vi "콜라자판기.vi"() -> ()   [LabVIEW 2014]
panel:
  out "그림 링":u16(ring)
  in  "종료":bool
  in  "반환":bool
  in  "구매":bool
  out "투입금액형":i32
  in  "동전":T1
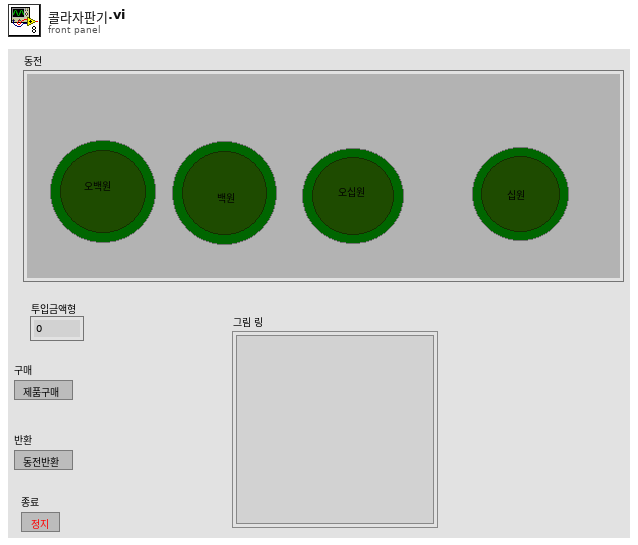
[diagram p1: front panel]
types:
  T1 = cluster{"오백원":bool, "백원":bool, "오십원":bool, "십원":bool}
  T2 = typedef "자판기.ctl" = enum16{"idle", "초기화", "종료", "구매", "반환"}
  T3 = enum8{"Enabled", "Disabled", "Disabled and Grayed Out"}
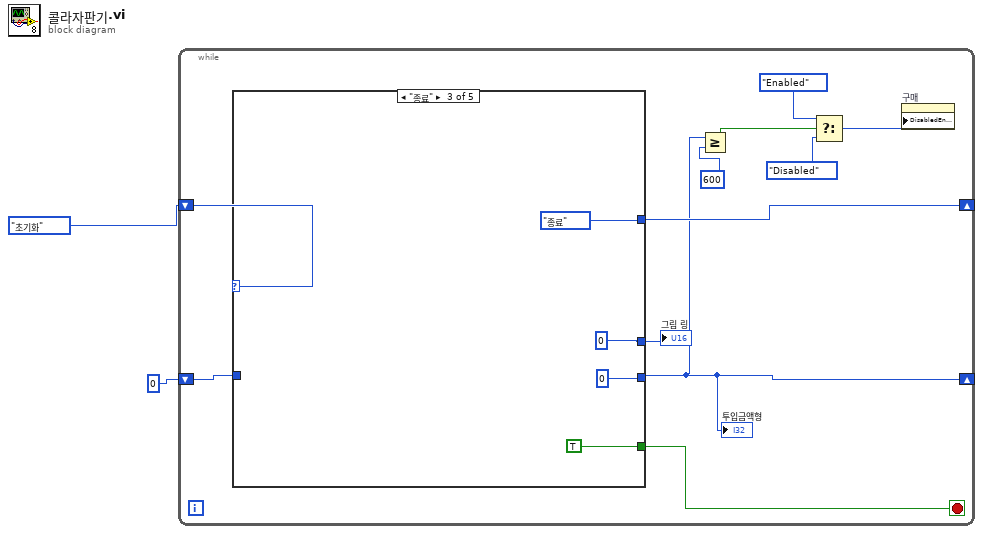
[diagram p0: block diagram]
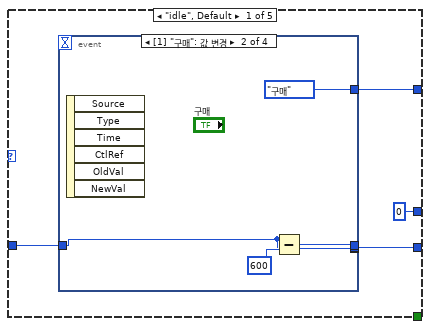
[diagram p2: hidden frame]
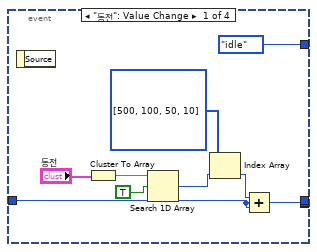
[diagram p3: hidden frame]
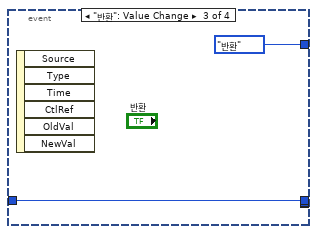
[diagram p4: hidden frame]
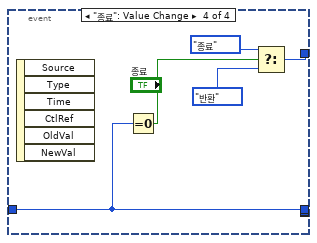
[diagram p5: hidden frame]
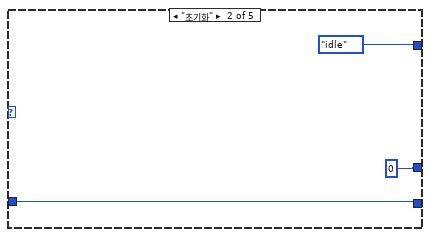
[diagram p6: hidden frame]
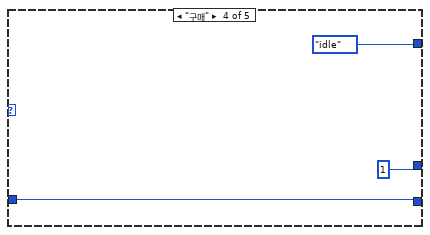
[diagram p7: hidden frame]
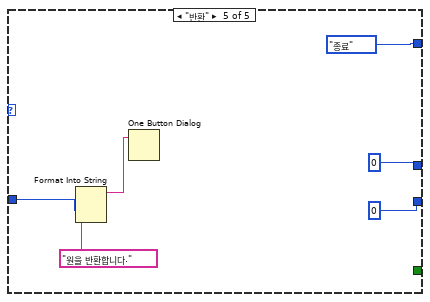
[diagram p8: hidden frame]
diagram:
  n1 = while {
    shift-right: [w12] -> _
    shift-left: 자판기."초기화" ("열거형") -> [w13]
    shift-right: [w9] -> _
    shift-left: 0 -> [w11]
    stop <- w3 stop-if-true
    n2 = case shown="\"종료\"" w13 {
      tunnel: [w17 자판기."idle" ("열거형") 자판기."종료" ("열거형") 자판기."idle" ("열거형") 자판기."종료" ("열거형")] -> w12
      tunnel: w11 -> [w14 w38 _ w45 w50]
      tunnel: [w16 w38 0 w45 0] -> w9
      tunnel: [u16 0 u16 0 u16 0 u16 1 u16 0] -> w10
      tunnel: [_ _ TRUE _ _] -> w3
      frame "idle", Default {
        n3 = event shown="[1] \"구매\": 값 변경" {
          selector: _ -> [_ _ _ _]
          dyn-events: _ -> [_ _ _ _]
          timeout: _ -> [_ _ _ _]
          tunnel: [자판기."idle" ("열거형") 자판기."구매" ("열거형") 자판기."반환" ("열거형") w37] -> w17
          tunnel: [w18 w27 _ _] -> _
          tunnel: [w19 w29 _ _] -> w16
          tunnel: [_ _ w31 w34] -> _
          tunnel: w14 -> [w18 w27 w31 w34]
          event "동전": Value Change {
            n4 = event-data() -> ()  [unwired: 1 in, 1 out]
            n5 = Cluster To Array(cluster="동전") -> (array=w23:bool[])
            n6 = Search 1D Array(1D array=w23, element=TRUE) -> (index of element=w22:i32)  [unwired: 1 in]
            n7 = Index Array(array=i32[] [500, 100, 50, 10], index=w22) -> (element=w20:i32)
            n8 = Add(x=w20, y=w18) -> (x+y=w19:i32)
          }
          event "구매": Value Change {
            n9 = event-data() -> ()  [unwired: 1 in, 6 out]
            n10 = Subtract(x=w27, y=600) -> (x-y=w29:i32)
          }
          event "반환": Value Change {
            n11 = event-data() -> ()  [unwired: 1 in, 6 out]
          }
          event "종료": Value Change {
            n12 = event-data() -> ()  [unwired: 1 in, 6 out]
            n13 = Equal To 0?(x=w34) -> (x = 0?=w33:bool)
            n14 = Select(t=자판기."종료" ("열거형"), s=w33, f=자판기."반환" ("열거형")) -> (s? t:f=w37:T2)
          }
        }
      }
      frame "초기화" {
      }
      frame "종료" {
      }
      frame "구매" {
      }
      frame "반환" {
        n15 = Format Into String(w50, "원을 반환합니다.") -> (resulting string=w49:string)  [unwired: 3 in, 1 out]
        n16 = One Button Dialog(message=w49) -> ()  [unwired: 1 in, 1 out]
      }
    }
    "그림 링" <- w10
    "투입금액형" <- w9
    n17 = Greater Or Equal?(x=w9, y=600) -> (x >= y?=w5:bool)
    n18 = Select(t=T3."Enabled" ("비활성화"), s=w5, f=T3."Disabled") -> (s? t:f=w4:T3)
    n19 = property on="구매" class="Bool"("DisabledEnum"=w4) -> ()  [unwired: 2 in, 2 out]
  }
